vi "Initialize Transfer.vi"(7 "id":i32, 8 "error in (no error)":errorcluster, 9 "convert (F)":bool, 10 "Buffers":refnum<class "Buffers.lvclass">, 11 "Transfer Configuration":refnum<class "Transfer Configuration.lvclass">) -> (0 "error out":errorcluster, 3 "Transfer out":refnum<class "Transfer.lvclass">)   [LabVIEW 2019, in "DSF Core.lvlib" / "Transfer.lvclass"]
uses:
  Transfer.lvclass
  Configuration/Core/Transfer/Transfer Configuration.lvclass
  Buffers/Buffers.lvclass
  Transfer.lvclass/Transfer.ctl
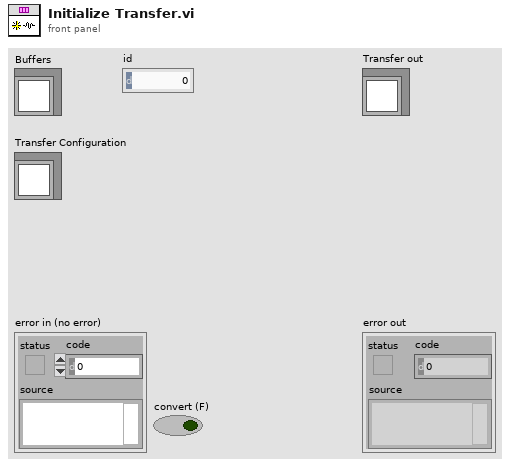
[diagram p1: front panel]
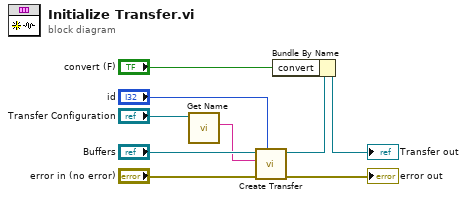
[diagram p0: block diagram]
diagram:
  n1 = call "Get Name.vi"("Transfer Configuration in"="Transfer Configuration") -> ("name"=w1:string)  [unwired: 8 in, 2 out]
  n2 = call "Create Transfer.vi"("id"="id", "error in (no error)"="error in (no error)", "name"=w1, "Buffers"="Buffers") -> ("error out"=→"error out":errorcluster, "Transfer out"=w5:refnum<class "Transfer.lvclass">)  [unwired: 6 in]
  n3 = Bundle By Name(cluster=w5, "convert"="convert (F)") -> (→"Transfer out":refnum<class "Transfer.lvclass">)
